vi "Read REFRESCOS Y PAPAS.vi"(8 "error in (no error)":errorcluster, 11 "MXN Actor in":refnum<class "MXN Actor.lvclass">) -> (0 "error out":errorcluster, 2 "REFRESCOS Y PAPAS":bool, 3 "MXN Actor out":refnum<class "MXN Actor.lvclass">)   [LabVIEW 2019, in "MXN Actor.lvlib" / "MXN Actor.lvclass"]
uses:
  MXN Actor.lvclass
  MXN Actor.lvclass/MXN Actor.ctl
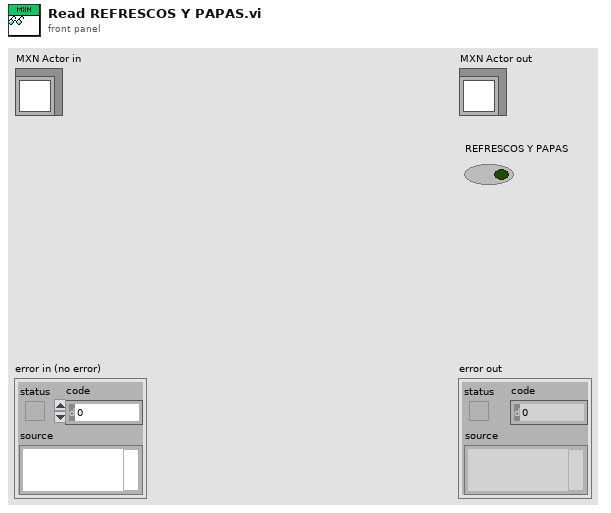
[diagram p1: front panel]
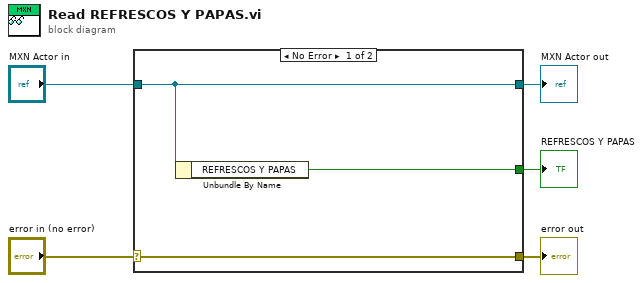
[diagram p0: block diagram]
diagram:
  n1 = case shown="No Error" "error in (no error)" {
    selector: "error in (no error)" -> [w8 w9]
    tunnel: [w8 w9] -> w4
    tunnel: [w7 w10] -> w2
    tunnel: "MXN Actor in" -> [w7 w10]
    tunnel: [w6 _] -> w1
    frame No Error {
      n2 = Unbundle By Name(w7) -> ("REFRESCOS Y PAPAS"=w6:bool)
    }
    frame Error {
    }
  }
  "error out" <- w4
  "MXN Actor out" <- w2
  "REFRESCOS Y PAPAS" <- w1
